vi "Setup Client.vi"(0 "WAMP Client in":refnum<class "WAMP Client.lvclass">, 7 "Realm":string, 9 "Address":string, 11 "error in (no error)":errorcluster) -> (4 "WAMP client out":refnum<class "WAMP Client.lvclass">, 15 "error out":errorcluster)   [LabVIEW 2020, in "wamplv.lvlib" / "WAMP Client.lvclass"]
doc: "Sets up the connection parameters of wamplv.If you are inheriting from wamplv, pass your child class to this VI for it to get setup properly.\n\nYou don't need to use this VI if you use `New Client.vi`."
uses:
  WAMP Client.lvclass
  <vilib>/LabVIEW Open Source Project/OpenURI/uri/URI.lvclass/URI.ctl
  Private/Comm Handlers/RawSocket TCP Handler/RawSocket TCP Handler.lvclass
  C:/local/wamplv/Private/Comm Handlers/TCPSocketBasedCommHandlerBase/TCPSocketBasedCommHandlerBase.lvclass
  API/TypeDefs/Transport Type.ctl
  Private/Comm Handlers/Websocket Handler/Websocket Handler.lvclass
  WAMP Client.lvclass/WAMP Client.ctl
  Private/Comm Handlers/TCPSocketBasedCommHandlerBase/TCPSocketBasedCommHandlerBase.lvclass
  C:/local/wamplv/Private/Comm Handlers/ICommHandler/ICommHandler.lvclass
  <vilib>/Utility/error.llb/Error Cluster From Error Code.vi
  <vilib>/ErrorRing/Error Ring.xnode
  <vilib>/LabVIEW Open Source Project/OpenURI/uri/URI.lvclass
panel:
  # "If you are inheriting from wamplv, pass your child class to this\nVI for it to get setup properly.\n\nDon't use this VI if you are using New Client.vi."
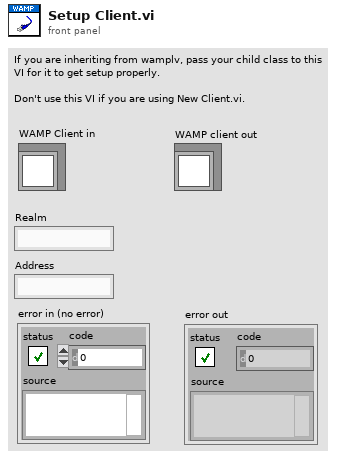
[diagram p1: front panel]
types:
  T1 = typedef "wamplv.lvlib/WAMP Client.lvclass/Transport Type.ctl" = enum16{"WebSocket", "RawSocket TCP"}
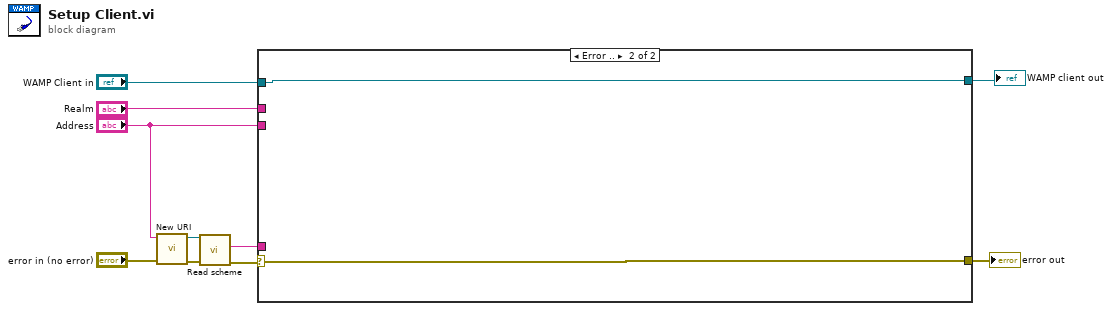
[diagram p0: block diagram]
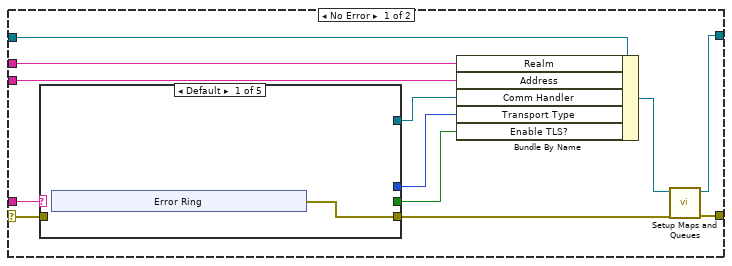
[diagram p2: hidden frame]
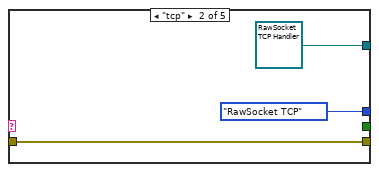
[diagram p3: hidden frame]
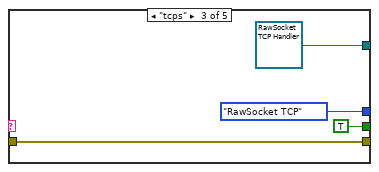
[diagram p4: hidden frame]
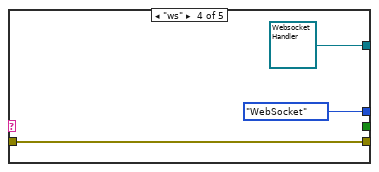
[diagram p5: hidden frame]
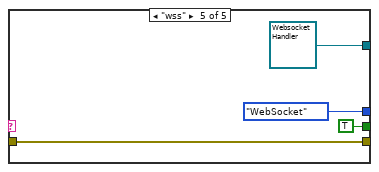
[diagram p6: hidden frame]
diagram:
  n1 = call <vilib>:"New URI.vi"("error in (no error)"="error in (no error)", "URI"="Address") -> ("error out"=w9:errorcluster, "URI"=w10:refnum<class "URI.lvclass">)  [unwired: 8 in]
  n2 = call <vilib>:"Read scheme.vi"("error in (no error)"=w9, "URI in"=w10) -> ("error out"=w8:errorcluster, "scheme"=w7:string)  [unwired: 7 in, 1 out]
  n3 = case shown="Error .." w8 {
    selector: w8 -> [w11 w43]
    tunnel: "Realm" -> [w18 _]
    tunnel: [w22 w42] -> w6
    tunnel: [w21 w43] -> w4
    tunnel: "Address" -> [w17 _]
    tunnel: w7 -> [w20 _]
    tunnel: "WAMP Client in" -> [w16 w42]
    frame No Error {
      n4 = case shown="Default" w20 {
        tunnel: [_ refnum<class "RawSocket TCP Handler.lvclass"> refnum ("wamplv.lvlib:RawSocket Handler.lvclass") refnum<class "RawSocket TCP Handler.lvclass"> refnum ("wamplv.lvlib:RawSocket Handler.lvclass") refnum<class "Websocket Handler.lvclass"> refnum ("Websocket Handler.lvclass") refnum<class "Websocket Handler.lvclass"> refnum ("Websocket Handler.lvclass")] -> w19
        tunnel: [w23 w28 w31 w35 w38] -> w13
        tunnel: [_ Transport_Type."RawSocket TCP" ("Transport Type") Transport_Type."RawSocket TCP" ("Transport Type") Transport_Type."WebSocket" ("Transport Type") Transport_Type."WebSocket" ("Transport Type")] -> w15
        tunnel: [_ _ TRUE ("Transport Options.Enable TLS?") _ TRUE ("Transport Options.Enable TLS?")] -> w14
        tunnel: w11 -> [_ w28 w31 w35 w38]
        frame Default {
          n5 = xnode "Error Ring"() -> ("error out"=w23:errorcluster)
        }
        frame "tcp" {
        }
        frame "tcps" {
        }
        frame "ws" {
        }
        frame "wss" {
        }
      }
      n6 = Bundle By Name(cluster=w16, "Realm"=w18, "Address"=w17, "Comm Handler"=w19, "Transport Type"=w15, "Enable TLS?"=w14) -> (w12:refnum<class "WAMP Client.lvclass">)
      n7 = call-dynamic "Setup Maps and Queues.vi"("error in (no error)"=w13, "WAMP Client in"=w12) -> ("error out"=w21:errorcluster, "WAMP Client out"=w22:refnum<class "WAMP Client.lvclass">)  [unwired: 8 in]
    }
    frame Error {
    }
  }
  "error out" <- w4
  "WAMP client out" <- w6
